vi "Loop_HW Camera.vi"() -> ()   [LabVIEW 2017, in "VisionSystem.lvlib"]
uses:
  VisionSystem.lvlib
  ENUM_HW_State.ctl
  Cluster_CMD to Vision.ctl
  Enum_ Field Targets.ctl
  ENUM_HW_Action.ctl
  Cluster_HW_Status.ctl
  <vilib>/vision/Image Controls.llb/IMAQ Image.ctl
  TypeDefs/Cluster_Camera Settings.ctl
  <vilib>/Rock Robotics/WPI/Camera/WPI_CameraImageSize.ctl
  <vilib>/Rock Robotics/WPI/Camera/WPI_CameraFrameRate.ctl
  <vilib>/Rock Robotics/WPI/Camera/WPI_CameraWhite Balance Values.ctl
  <vilib>/Rock Robotics/WPI/Camera/WPI_CameraExposure Values.ctl
  <vilib>/Rock Robotics/WPI/Camera/WPI_CameraDevRef.ctl
  Global_CMD Data.vi
  Globals/Global_STOP.vi
  Global_HW Status.vi
  <vilib>/vision/driver/NI_Vision_Acquisition_Software.lvlib
panel:
  in  "Clear error":bool
  in  "Reset Camera":bool
  in  "Reset Camera":bool
  out "cycle time (s)":dbl
  in  "Cam 1 Setings":T1={"Image Size"=enum."320x240", "Frame Rate (fps)"=35, "White Balance"=enum."Custom", "Exposure"=enum."Auto", "Exposure (%)"=0.0, "Brightness"=72, "Sharpness"=0, "Saturation"=0} {"Saturation" min=0 max=100 step=1; "Sharpness" min=0 max=100 step=1; "Brightness" min=0 max=100 step=1; "Exposure (%)" min=0.0 max=100.0 step=1.0}
  out "Error":errorcluster[](array[cluster])
  in  "Restore Settings":bool
  in  "Save Settings":bool
  in  "Cam 0 Setings":T1={"Image Size"=enum."320x240", "Frame Rate (fps)"=20, "White Balance"=enum."Auto", "Exposure"=enum."Auto", "Exposure (%)"=0.0, "Brightness"=0, "Sharpness"=0, "Saturation"=0} {"Saturation" min=0 max=100 step=1; "Sharpness" min=0 max=100 step=1; "Brightness" min=0 max=100 step=1; "Exposure (%)" min=0.0 max=100.0 step=1.0}
  out "Cam Array":T6(array[cluster]) {"BusType" format="%x"; "SerialNumberLow" format="%.0x"; "SerialNumberHigh" format="%.0x"}
  out "Image":T7(plugin-control)
  in  "Show Image":bool
  out "HW Status_OUT":T8 {"Cam Setings"."Saturation" min=0 max=100 step=1; "Cam Setings"."Sharpness" min=0 max=100 step=1; "Cam Setings"."Brightness" min=0 max=100 step=1; "Cam Setings"."Exposure (%)" min=0.0 max=100.0 step=1.0}
  out "Action":T11
  out "CMD_Camera":T12
  out "Current State":T13
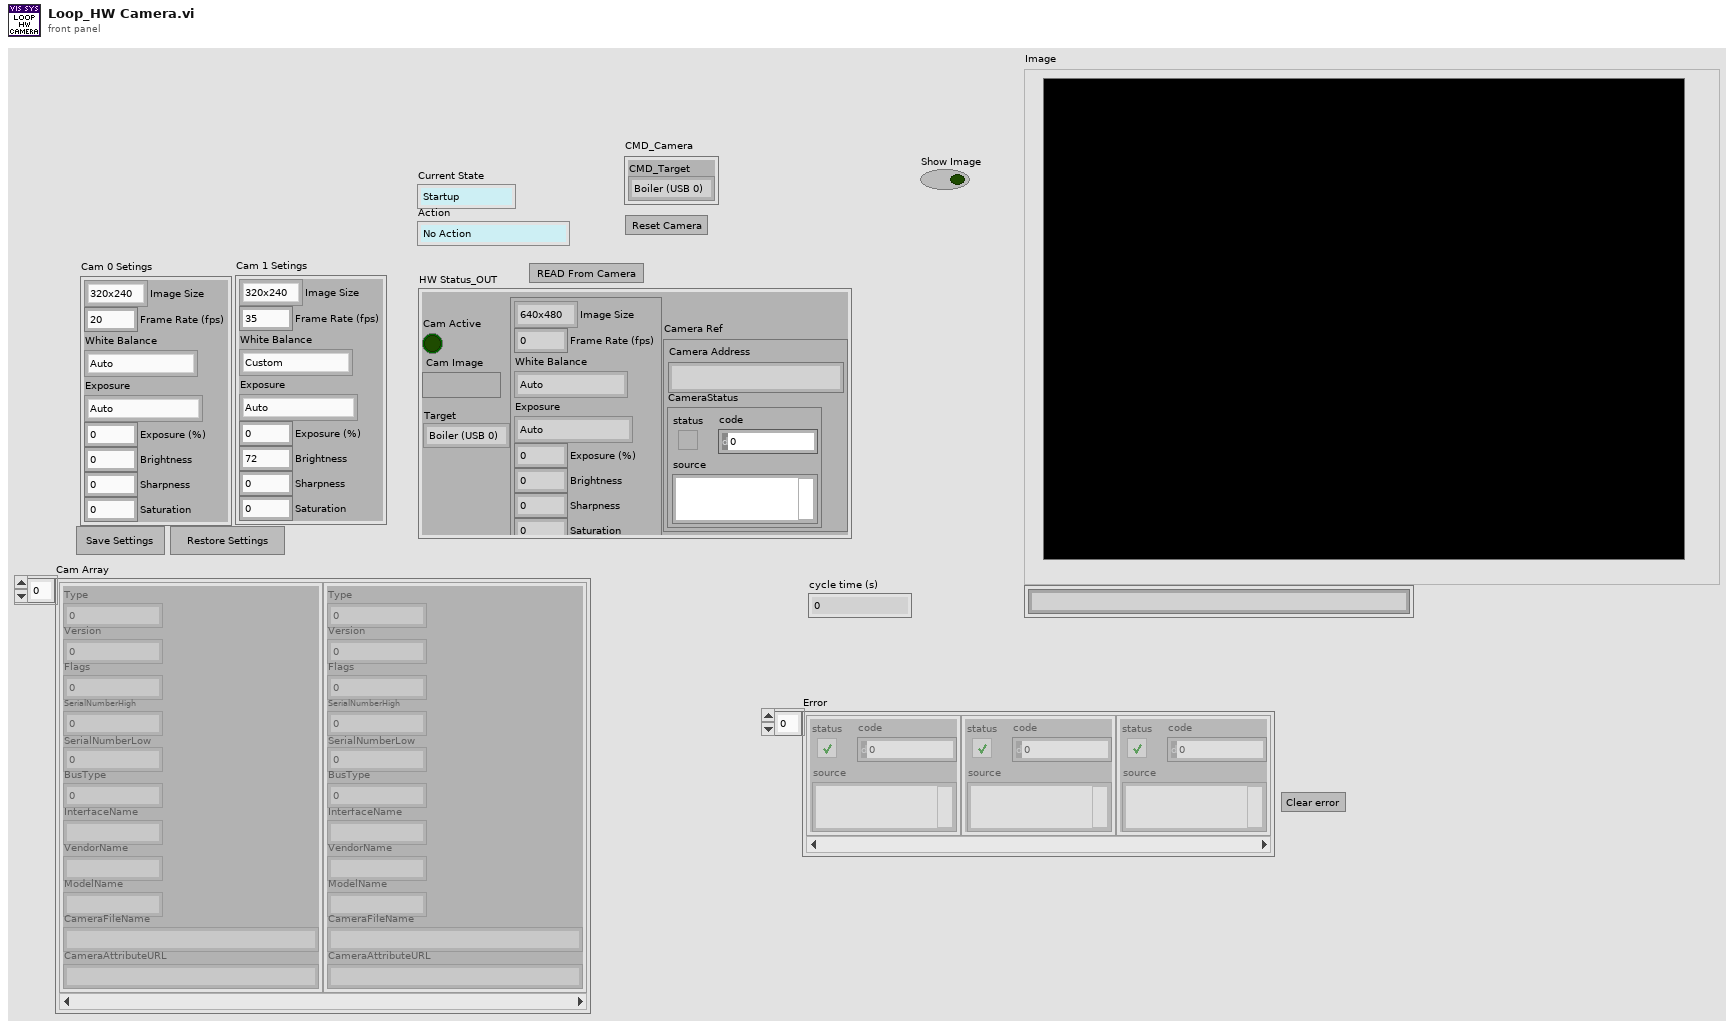
[diagram p1: front panel]
types:
  T1 = typedef "Cluster_Camera Settings.ctl" = cluster{"Image Size":T2, "Frame Rate (fps)":T3, "White Balance":T4, "Exposure":T5, "Exposure (%)":dbl, "Brightness":i32, "Sharpness":i32, "Saturation":i32}
  T2 = typedef "WPI_CameraImageSize.ctl" = enum16{"640x480", "320x240", "160x120", "Custom"}
  T3 = typedef "WPI_CameraFrameRate.ctl" = u32
  T4 = typedef "WPI_CameraWhite Balance Values.ctl" = enum16{"Auto", "Fixed indoor", "Fixed outdoor 1", "Fixed outdoor 2", "Fixed fluorescent 1", "Fixed fluorescent 2", "Hold current", "Custom"}
  T5 = typedef "WPI_CameraExposure Values.ctl" = enum16{"Auto", "Flicker-free 50 Hz", "Flicker-free 60 Hz", "Hold current", "Custom"}
  T6 = cluster{"Type":u32, "Version":u32, "Flags":u32, "SerialNumberHigh":u32, "SerialNumberLow":u32, "BusType":u32, "InterfaceName":string, "VendorName":string, "ModelName":string, "CameraFileName":string, "CameraAttributeURL":string}[]
  T7 = typedef "IMAQ Image.ctl" = refnum<image>
  T8 = typedef "VisionSystem.lvlib/Cluster_HW_Status.ctl" = cluster{"Cam Active":bool, "Cam Image":T7, "Cam Setings":T1, "Target":T9, "Camera Ref":T10}
  T9 = typedef "VisionSystem.lvlib/Enum_ Field Targets.ctl" = enum16{"Boiler (USB 0)", "Rope (USB 1)"}
  T10 = typedef "WPI_CameraDevRef.ctl" = cluster{"Camera Address":string, "CameraStatus":errorcluster}
  T11 = typedef "VisionSystem.lvlib/ENUM_HW_Action.ctl" = enum16{"No Action", "Reset Time", "Open Cam 0", "Open Cam 1", "Stop Camera", "Start Camera", "Acquire Camera", "Close Camera", "Read Avalable Cams", "Save Settings to File", "Restore Settings from File", "Open Image", "Close Image", "Set  Camera", "Read Cam Settings"}
  T12 = typedef "VisionSystem.lvlib/Cluster_CMD to Vision.ctl" = cluster{"CMD_Target":T9}
  T13 = typedef "VisionSystem.lvlib/ENUM_HW_State.ctl" = enum16{"Startup", "Idle", "Acquire", "Shutdown", "Setting"}
  T14 = cluster{"Actions":T11[], "State":T13, "Current Time":timestamp, "Start Time":timestamp, "Loop Time (ms)":u32, "CMD_HW":T12, "HW Status_OUT":T8, "Cam  Array":cluster{"Type":u32, "Version":u32, "Flags":u32, "SerialNumberHigh":u32, "SerialNumberLow":u32, "BusType":u32, "InterfaceName":string, "VendorName":string, "ModelName":string, "CameraFileName":string, "CameraAttributeURL":string}[], "Error ":errorcluster[], "Cam 0 Setings":T1, "Cam 1 Setings":T1, "Camera Readings":T1}
  T15 = typedef "Image Type" = u32
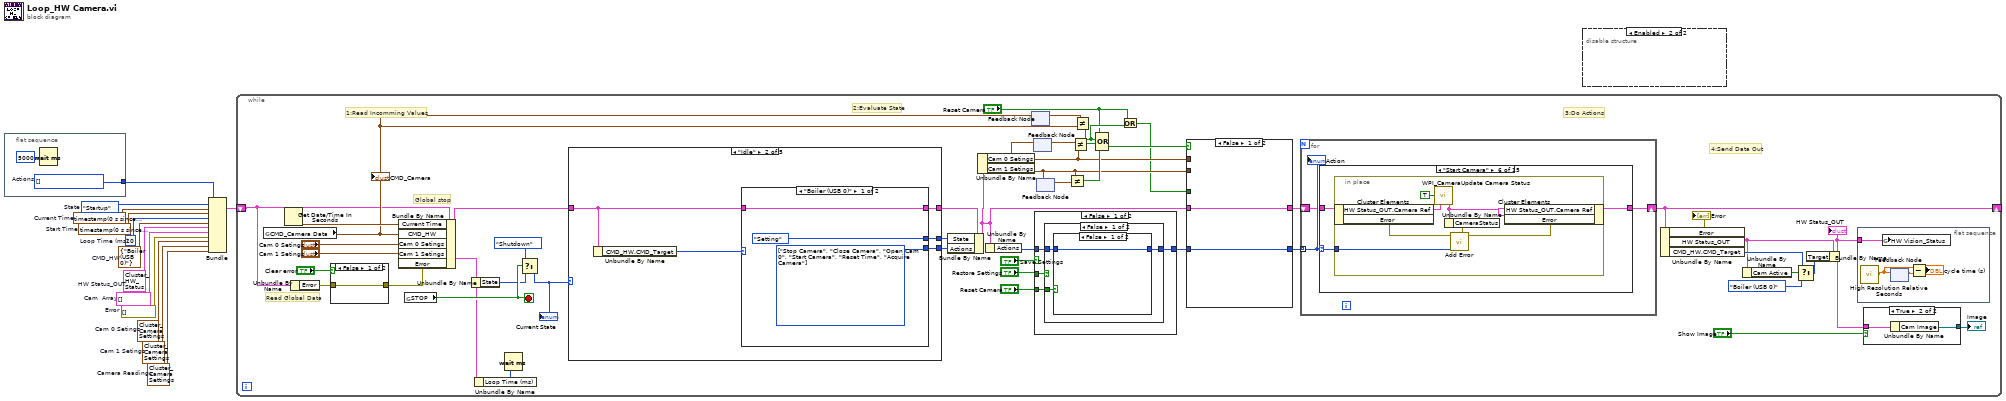
[diagram p0: block diagram]
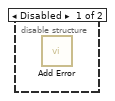
[diagram p2: hidden frame]
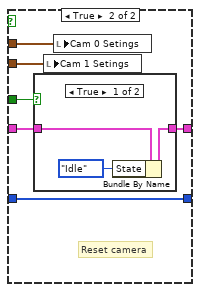
[diagram p4: hidden frame]
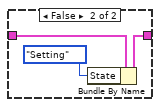
[diagram p5: hidden frame]
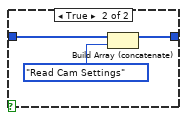
[diagram p6: hidden frame]
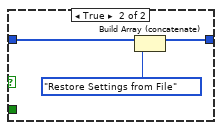
[diagram p7: hidden frame]
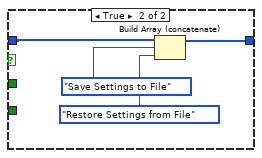
[diagram p8: hidden frame]
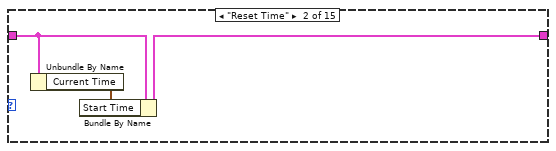
[diagram p11: hidden frame]
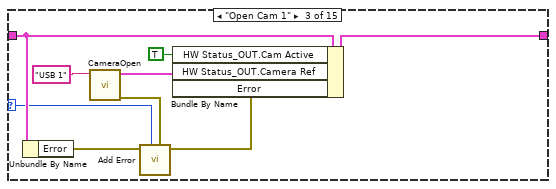
[diagram p12: hidden frame]
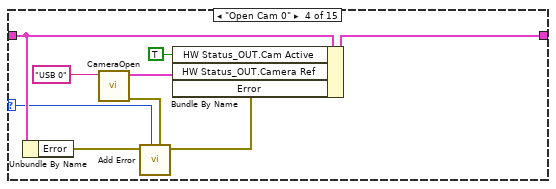
[diagram p13: hidden frame]
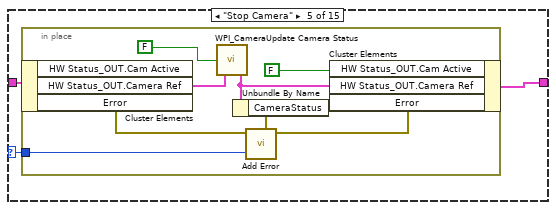
[diagram p14: hidden frame]
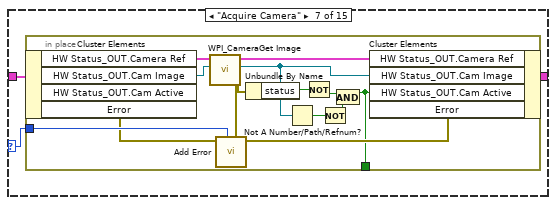
[diagram p15: hidden frame]
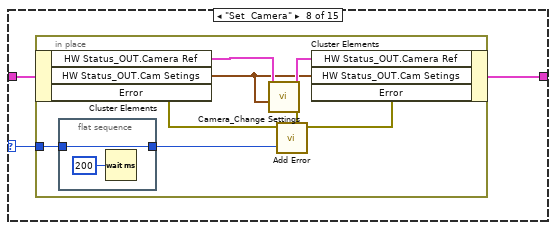
[diagram p16: hidden frame]
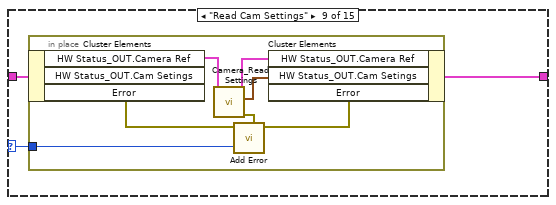
[diagram p17: hidden frame]
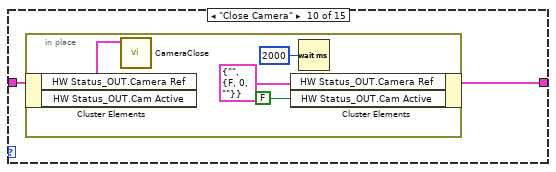
[diagram p18: hidden frame]
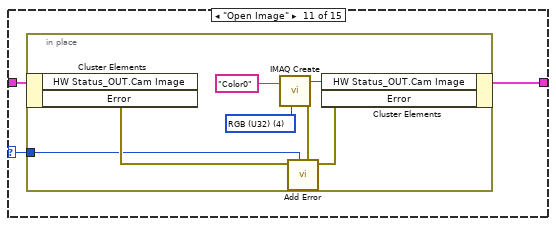
[diagram p19: hidden frame]
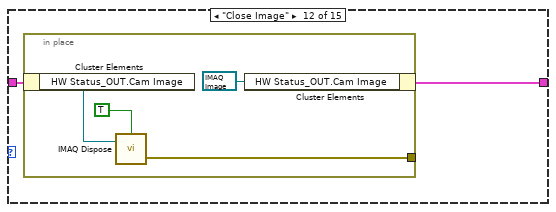
[diagram p20: hidden frame]
diagram:
  w1 = T1 {"Image Size"=enum."640x480", "Frame Rate (fps)"=20, "White Balance"=enum."Fixed fluorescent 1", "Exposure"=enum."Flicker-free 60 Hz", "Exposure (%)"=20.0, "Brightness"=0, "Sharpness"=0, "Saturation"=40}  # Camera Readings
  w2 = T1 {"Image Size"=enum."640x480", "Frame Rate (fps)"=0, "White Balance"=enum."Auto", "Exposure"=enum."Auto", "Exposure (%)"=0.0, "Brightness"=0, "Sharpness"=0, "Saturation"=0}  # Cam 1 Setings
  w3 = T1 {"Image Size"=enum."640x480", "Frame Rate (fps)"=0, "White Balance"=enum."Auto", "Exposure"=enum."Auto", "Exposure (%)"=0.0, "Brightness"=0, "Sharpness"=0, "Saturation"=0}  # Cam 0 Setings
  w4 = errorcluster[] []  # Error
  w5 = T6 []  # Cam  Array
  w6 = T8 {"Cam Active"=FALSE, "Cam Image"=refnum, "Cam Setings"={"Image Size"=enum."640x480", "Frame Rate (fps)"=0, "White Balance"=enum."Auto", "Exposure"=enum."Auto", "Exposure (%)"=0.0, "Brightness"=0, "Sharpness"=0, "Saturation"=0}, "Target"=enum."Boiler (USB 0)", "Camera Ref"={"Camera Address"="", "CameraStatus"={"status"=FALSE, "code"=0, "source"=""}}}  # HW Status_OUT
  w7 = T12 {"CMD_Target"=enum."Boiler (USB 0)"}  # CMD_HW
  w8 = u32 20  # Loop Time (ms)
  w10 = timestamp(0 s since 1904-01-01)  # Start Time
  w11 = timestamp(0 s since 1904-01-01)  # Current Time
  w12 = ENUM_HW_State."Startup"  # State
  n1 = flat-sequence {
    tunnel: [w15] -> w9
    frame #0 {
      w15 = T11[] [] items=["No Action", "Reset Time", "Open Cam 0", "Open Cam 1", "Stop Camera", "Start Camera", "Acquire Camera", "Close Camera", "Read Avalable Cams", "Save Settings to File", "Restore Settings from File", "Open Image", "Close Image", "Set  Camera", "Read Cam Settings"]  # Actions
      n2 = Wait (ms)(milliseconds to wait=u32 5000) -> ()  [unwired: 1 out]
    }
  }
  n3 = Bundle("Actions"=w9, "State"=w12, "Current Time"=w11, "Start Time"=w10, "Loop Time (ms)"=w8, "CMD_HW"=w7, "HW Status_OUT"=w6, "Cam  Array"=w5, "Error"=w4, "Cam 0 Setings"=w3, "Cam 1 Setings"=w2, "Camera Readings"=w1) -> (w13:T14)  [unwired: 1 in]
  n4 = while {
    shift-right: [w23] -> _
    shift-left: w13 -> [w22]
    stop <- w56 stop-if-true
    # "Read Global Data"
    # "1:Read Incomming Values"
    # "2:Evaluate State"
    # "3:Do Actions"
    # "4:Send Data Out"
    # "Global stop"
    n5 = global read "Global_CMD Data.vi" "CMD_Camera Data"() -> (w25:T12)
    "CMD_Camera" <- w25
    n6 = Get Date/Time In Seconds() -> (seconds since 1Jan1904=w60:timestamp)
    n7 = Unbundle By Name(w22) -> ("Error"=w20:errorcluster[])
    n8 = case shown="False" "Clear error" {
      tunnel: [w62 _] -> w19
      tunnel: w20 -> [w62 _]
      frame False {
      }
      frame True {
      }
    }
    n9 = Bundle By Name(cluster=w22, "Current Time"=w60, "CMD_HW"=w25, "Cam 0 Setings"="Cam 0 Setings", "Cam 1 Setings"="Cam 1 Setings", "Error"=w19) -> (w51:T14)
    n10 = global read "Global_Stop.vi" "STOP"() -> (w56:bool)
    n11 = Unbundle By Name(w51) -> ("State"=w54:T13)
    n12 = Unbundle By Name(w51) -> ("Loop Time (ms)"=w52:u32)
    n13 = Wait (ms)(milliseconds to wait=w52) -> ()  [unwired: 1 out]
    n14 = Select(t=ENUM_HW_State."Shutdown" ("State"), s=w56, f=w54) -> (s? t:f=w53:T13)
    "Current State" <- w53
    n15 = case shown="\"Idle\"" w53 {
      tunnel: w51 -> [w247 w251 w263 w291 w294]
      tunnel: [w247 w250 w262 w291 w294] -> w59
      tunnel: [ENUM_HW_State."Idle" ("State") w249 w261 ENUM_HW_State."Acquire" ("State") ENUM_HW_State."Shutdown" ("State")] -> w58
      tunnel: [w246 w248 w260 w289 w292] -> w57
      frame "Startup" {
        w246 = T11[] [enum."Read Avalable Cams", enum."Restore Settings from File", enum."Open Image", enum."Close Camera"] items=["No Action", "Reset Time", "Open Cam 0", "Open Cam 1", "Stop Camera", "Start Camera", "Acquire Camera", "Close Camera", "Read Avalable Cams", "Save Settings to File", "Restore Settings from File", "Open Image", "Close Image", "Set  Camera", "Read Cam Settings"] ("Actions")
      }
      frame "Idle" {
        n16 = Unbundle By Name(w251) -> ("CMD_HW.CMD_Target"=w252:T9)
        n17 = case shown="\"Boiler (USB 0)\"" w252 {
          tunnel: w251 -> [w253 w256]
          tunnel: [w253 w256] -> w250
          tunnel: [ENUM_HW_State."Setting" ("State") ENUM_HW_State."Setting" ("State")] -> w249
          tunnel: [w254 w257] -> w248
          frame "Boiler (USB 0)" {
            w254 = T11[] [enum."Stop Camera", enum."Close Camera", enum."Open Cam 0", enum."Start Camera", enum."Reset Time", enum."Acquire Camera"] items=["No Action", "Reset Time", "Open Cam 0", "Open Cam 1", "Stop Camera", "Start Camera", "Acquire Camera", "Close Camera", "Read Avalable Cams", "Save Settings to File", "Restore Settings from File", "Open Image", "Close Image", "Set  Camera", "Read Cam Settings"] ("Actions")
          }
          frame "Rope (USB 1)" {
            w257 = T11[] [enum."Stop Camera", enum."Close Camera", enum."Open Cam 1", enum."Start Camera", enum."Reset Time"] items=["No Action", "Reset Time", "Open Cam 0", "Open Cam 1", "Stop Camera", "Start Camera", "Acquire Camera", "Close Camera", "Read Avalable Cams", "Save Settings to File", "Restore Settings from File", "Open Image", "Close Image", "Set  Camera", "Read Cam Settings"] ("Actions")
          }
        }
      }
      frame "Setting" {
        n18 = Unbundle By Name(w263) -> ("HW Status_OUT.Cam Active"=w259:bool, "CMD_HW.CMD_Target"=w264:T9)
        n19 = case shown="False" w259 {
          tunnel: w264 -> [_ w278]
          tunnel: w263 -> [w273 w277]
          tunnel: [w273 w276] -> w262
          tunnel: [w265 w275] -> w261
          tunnel: [_ w274] -> w260
          frame False {
            n20 = Unbundle By Name(w273) -> ("Current Time"=w272:timestamp, "Start Time"=w271:timestamp)
            n21 = Subtract(x=w272, y=w271) -> (x-y=w270:dbl)
            n22 = Greater Or Equal?(x=w270, y=2.0) -> (x >= y?=w268:bool)
            n23 = Select(t=ENUM_HW_State."Idle" ("State"), s=w268, f=ENUM_HW_State."Setting" ("State")) -> (s? t:f=w265:T13)
          }
          frame True {
            n24 = case shown="\"Rope (USB 1)\"" w278 {
              tunnel: w277 -> [w282 w287]
              tunnel: [w281 w286] -> w276
              tunnel: [ENUM_HW_State."Acquire" ("State") ENUM_HW_State."Acquire" ("State")] -> w275
              tunnel: [w279 w284] -> w274
              frame "Rope (USB 1)" {
                w279 = T11[] [enum."Set  Camera", enum."Read Cam Settings", enum."Acquire Camera"] items=["No Action", "Reset Time", "Open Cam 0", "Open Cam 1", "Stop Camera", "Start Camera", "Acquire Camera", "Close Camera", "Read Avalable Cams", "Save Settings to File", "Restore Settings from File", "Open Image", "Close Image", "Set  Camera", "Read Cam Settings"] ("Actions")
                n25 = Unbundle By Name(w282) -> ("Cam 1 Setings"=w280:T1)
                n26 = Bundle By Name(cluster=w282, "HW Status_OUT.Cam Setings"=w280) -> (w281:T14)
              }
              frame "Boiler (USB 0)" {
                w284 = T11[] [enum."Set  Camera", enum."Read Cam Settings", enum."Acquire Camera"] items=["No Action", "Reset Time", "Open Cam 0", "Open Cam 1", "Stop Camera", "Start Camera", "Acquire Camera", "Close Camera", "Read Avalable Cams", "Save Settings to File", "Restore Settings from File", "Open Image", "Close Image", "Set  Camera", "Read Cam Settings"] ("Actions")
                n27 = Unbundle By Name(w287) -> ("Cam 0 Setings"=w285:T1)
                n28 = Bundle By Name(cluster=w287, "HW Status_OUT.Cam Setings"=w285) -> (w286:T14)
              }
            }
          }
        }
      }
      frame "Acquire" {
        w289 = T11[] [enum."Acquire Camera"] items=["No Action", "Reset Time", "Open Cam 0", "Open Cam 1", "Stop Camera", "Start Camera", "Acquire Camera", "Close Camera", "Read Avalable Cams", "Save Settings to File", "Restore Settings from File", "Open Image", "Close Image", "Set  Camera", "Read Cam Settings"] ("Actions")
      }
      frame "Shutdown" {
        w292 = T11[] [enum."Save Settings to File", enum."Stop Camera", enum."Close Camera", enum."Close Image"] items=["No Action", "Reset Time", "Open Cam 0", "Open Cam 1", "Stop Camera", "Start Camera", "Acquire Camera", "Close Camera", "Read Avalable Cams", "Save Settings to File", "Restore Settings from File", "Open Image", "Close Image", "Set  Camera", "Read Cam Settings"] ("Actions")
      }
    }
    n29 = Bundle By Name(cluster=w59, "State"=w58, "Actions"=w57) -> (w35:T14)
    n30 = Unbundle By Name(w35) -> ("Cam 0 Setings"=w27:T1, "Cam 1 Setings"=w28:T1)
    n31 = Unbundle By Name(w35) -> ("Actions"=w61:T11[])
    n32 = feedback #1() -> (w26:T12)  [unwired: 1 in]
    n33 = feedback-in #1(w25) -> ()
    n34 = feedback #2() -> (w42:T1)  [unwired: 1 in]
    n35 = feedback-in #2(w27) -> ()
    n36 = case shown="False" "Save Settings" {
      tunnel: w61 -> [w84 w98]
      tunnel: [w83 w97] -> w39
      tunnel: "Restore Settings" -> [w82 _]
      tunnel: "Reset Camera" -> [w81 _]
      frame False {
        n37 = case shown="False" w82 {
          tunnel: w84 -> [w86 w94]
          tunnel: [w85 w93] -> w83
          tunnel: w81 -> [w87 _]
          frame False {
            n38 = case shown="False" w87 {
              tunnel: w86 -> [w88 w91]
              tunnel: [w88 w90] -> w85
              frame False {
              }
              frame True {
                n39 = Build Array (concatenate)(w91, ENUM_HW_Action."Read Cam Settings" ("Action")) -> (w90:T11[])
              }
            }
          }
          frame True {
            n40 = Build Array (concatenate)(w94, ENUM_HW_Action."Restore Settings from File" ("Action")) -> (w93:T11[])
          }
        }
      }
      frame True {
        n41 = Build Array (concatenate)(w98, ENUM_HW_Action."Save Settings to File" ("Action"), ENUM_HW_Action."Restore Settings from File" ("Action")) -> (w97:T11[])
      }
    }
    n42 = feedback-in #3(w28) -> ()
    n43 = feedback #3() -> (w43:T1)  [unwired: 1 in]
    n44 = Not Equal?(x=w28, y=w43) -> (x != y?=w40:bool)
    n45 = Not Equal?(x=w42, y=w27) -> (x != y?=w41:bool)
    n46 = Not Equal?(x=w26, y=w25) -> (x != y?=w18:bool)
    n47 = Compound Arithmetic op=OR("Reset Camera", w18, w41, w40) -> (w37:bool)
    n48 = Or(x="Reset Camera", y=w18) -> (x .or. y?=w16:bool)
    n49 = case shown="False" w37 {
      tunnel: w39 -> [w68 w74]
      tunnel: [w68 w74] -> w38
      tunnel: [w67 w72] -> w36
      tunnel: w35 -> [w67 w73]
      tunnel: w28 -> [_ w71]
      tunnel: w27 -> [_ w70]
      tunnel: w16 -> [_ w69]
      frame False {
      }
      frame True {
        # "Reset camera"
        n50 = case shown="True" w69 {
          tunnel: w73 -> [w77 w80]
          tunnel: [w76 w79] -> w72
          frame True {
            n51 = Bundle By Name(cluster=w77, "State"=ENUM_HW_State."Idle") -> (w76:T14)
          }
          frame False {
            n52 = Bundle By Name(cluster=w80, "State"=ENUM_HW_State."Setting") -> (w79:T14)
          }
        }
        n53 = local write "Cam 1 Setings"(w71) -> ()
        n54 = local write "Cam 0 Setings"(w70) -> ()
      }
    }
    n55 = for {
      tunnel: w38 -> [w103] mode=indexing
      shift-right: [w102] -> w23
      shift-left: w36 -> [w101]
      n56 = case shown="\"Start Camera\"" w103 {
        selector: w103 -> [_ _ w111 w120 w126 w137 w149 w163 w176 _ w192 _ w208 w215 w230]
        tunnel: w101 -> [w104 w107 w113 w122 w128 w139 w148 w165 w178 w187 w194 w203 w212 w217 w232]
        tunnel: [w104 w106 w115 w124 w127 w138 w147 w164 w177 w186 w193 w202 w213 w216 w231] -> w102
        frame "No Action" {
        }
        frame "Reset Time" {
          n57 = Unbundle By Name(w107) -> ("Current Time"=w105:timestamp)
          n58 = Bundle By Name(cluster=w107, "Start Time"=w105) -> (w106:T14)
        }
        frame "Open Cam 1" {
          n59 = Unbundle By Name(w113) -> ("Error"=w112:errorcluster[])
          n60 = call "CameraOpen.vi"("Camera Address"="USB 1" ("format string")) -> ("error out"=w109:errorcluster, "CameraDevRef"=w114:T10)  [unwired: 1 in, 8 out]
          n61 = call "Add Error.vi"("Error"=w109, "Action"=w111, "Error list"=w112) -> ("Error list Out"=w110:errorcluster[])  [unwired: 8 in]
          n62 = Bundle By Name(cluster=w113, "HW Status_OUT.Cam Active"=TRUE, "HW Status_OUT.Camera Ref"=w114, "Error"=w110) -> (w115:T14)
        }
        frame "Open Cam 0" {
          n63 = Unbundle By Name(w122) -> ("Error"=w121:errorcluster[])
          n64 = call "CameraOpen.vi"("Camera Address"="USB 0" ("format string")) -> ("error out"=w118:errorcluster, "CameraDevRef"=w123:T10)  [unwired: 1 in, 8 out]
          n65 = call "Add Error.vi"("Error"=w118, "Action"=w120, "Error list"=w121) -> ("Error list Out"=w119:errorcluster[])  [unwired: 8 in]
          n66 = Bundle By Name(cluster=w122, "HW Status_OUT.Cam Active"=TRUE, "HW Status_OUT.Camera Ref"=w123, "Error"=w119) -> (w124:T14)
        }
        frame "Stop Camera" {
          n67 = in-place {
            in-place-border: w126 -> [w134]
            n68 = in-place-cluster #4(w128) -> ("HW Status_OUT.Camera Ref"=w135:T10, "Error"=w133:errorcluster[])  [unwired: 1 out]
            n69 = call <vilib>:"WPI_CameraUpdate Camera Status.vi"("CameraDevRef In"=w135, "Enable Vision"=FALSE) -> ("CameraDevRef Out"=w131:T10)  [unwired: 3 in]
            n70 = Unbundle By Name(w131) -> ("CameraStatus"=w130:errorcluster)
            n71 = call "Add Error.vi"("Error"=w130, "Action"=w134, "Error list"=w133) -> ("Error list Out"=w132:errorcluster[])  [unwired: 8 in]
            n72 = in-place-cluster #4("HW Status_OUT.Cam Active"=FALSE, "HW Status_OUT.Camera Ref"=w131, "Error"=w132) -> (w127:T14)
          }
        }
        frame "Start Camera" {
          n73 = in-place {
            in-place-border: w137 -> [w144]
            n74 = in-place-cluster #5(w139) -> ("HW Status_OUT.Camera Ref"=w145:T10, "Error"=w143:errorcluster[])
            n75 = call <vilib>:"WPI_CameraUpdate Camera Status.vi"("CameraDevRef In"=w145, "Enable Vision"=TRUE) -> ("CameraDevRef Out"=w141:T10)  [unwired: 3 in]
            n76 = Unbundle By Name(w141) -> ("CameraStatus"=w140:errorcluster)
            n77 = call "Add Error.vi"("Error"=w140, "Action"=w144, "Error list"=w143) -> ("Error list Out"=w142:errorcluster[])  [unwired: 8 in]
            n78 = in-place-cluster #5("HW Status_OUT.Camera Ref"=w141, "Error"=w142) -> (w138:T14)
          }
        }
        frame "Acquire Camera" {
          n79 = in-place {
            in-place-border: w149 -> [w159]
            in-place-border: [w150] -> _
            n80 = in-place-cluster #6(w148) -> ("HW Status_OUT.Camera Ref"=w162:T10, "HW Status_OUT.Cam Image"=w160:T7, "Error"=w158:errorcluster[])  [unwired: 1 out]
            n81 = call <vilib>:"WPI_CameraGet Image.vi"("Image"=w160, "CameraDevRef"=w162) -> ("error out"=w156:errorcluster, "Image Out"=w153:T7, "CameraDevRef Out"=w161:T10)  [unwired: 7 in]
            n82 = call "Add Error.vi"("Error"=w156, "Action"=w159, "Error list"=w158) -> ("Error list Out"=w157:errorcluster[])  [unwired: 8 in]
            n83 = Unbundle By Name(w156) -> ("status"=w155:bool)
            n84 = Not A Number/Path/Refnum?(number/path/refnum=w153) -> (NaN/Path/Refnum?=w152:bool)
            n85 = Not(x=w155) -> (.not. x?=w154:bool)
            n86 = Not(x=w152) -> (.not. x?=w151:bool)
            n87 = And(x=w154, y=w151) -> (x .and. y?=w150:bool)
            n88 = in-place-cluster #6("HW Status_OUT.Camera Ref"=w161, "HW Status_OUT.Cam Image"=w153, "HW Status_OUT.Cam Active"=w150, "Error"=w157) -> (w147:T14)
          }
        }
        frame "Set  Camera" {
          n89 = in-place {
            in-place-border: w163 -> [w167]
            n90 = in-place-cluster #7(w165) -> ("HW Status_OUT.Camera Ref"=w171:T10, "HW Status_OUT.Cam Setings"=w168:T1, "Error"=w173:errorcluster[])
            n91 = flat-sequence {
              tunnel: [w174] -> w166
              tunnel: w167 -> [w174]
              frame #0 {
                n92 = Wait (ms)(milliseconds to wait=u32 200) -> ()  [unwired: 1 out]
              }
            }
            n93 = call "Camera_Change Settings.vi"("Camera Settings"=w168, "CameraDevRef"=w171) -> ("Error Out"=w169:errorcluster, "CameraDevRef Out"=w170:T10)  [unwired: 8 in]
            n94 = call "Add Error.vi"("Error"=w169, "Action"=w166, "Error list"=w173) -> ("Error list Out"=w172:errorcluster[])  [unwired: 8 in]
            n95 = in-place-cluster #7("HW Status_OUT.Camera Ref"=w170, "HW Status_OUT.Cam Setings"=w168, "Error"=w172) -> (w164:T14)
          }
        }
        frame "Read Cam Settings" {
          n96 = in-place {
            in-place-border: w176 -> [w185]
            n97 = in-place-cluster #8(w178) -> ("HW Status_OUT.Camera Ref"=w182:T10, "Error"=w184:errorcluster[])  [unwired: 1 out]
            n98 = call "Camera_Read Settings.vi"("CameraDevRef"=w182) -> ("Error Out"=w180:errorcluster, "Camera Settings"=w179:T1, "CameraDevRef Out"=w181:T10)  [unwired: 8 in]
            n99 = call "Add Error.vi"("Error"=w180, "Action"=w185, "Error list"=w184) -> ("Error list Out"=w183:errorcluster[])  [unwired: 8 in]
            n100 = in-place-cluster #8("HW Status_OUT.Camera Ref"=w181, "HW Status_OUT.Cam Setings"=w179, "Error"=w183) -> (w177:T14)
          }
        }
        frame "Close Camera" {
          n101 = in-place {
            n102 = in-place-cluster #9(w187) -> ("HW Status_OUT.Camera Ref"=w191:T10)  [unwired: 1 out]
            n103 = call "CameraClose.vi"("CameraDevRef"=w191) -> ()  [unwired: 10 in, 1 out]
            n104 = in-place-cluster #9("HW Status_OUT.Camera Ref"=T10 {"Camera Address"="", "CameraStatus"={"status"=FALSE, "code"=0, "source"=""}} ("Cam Ref"), "HW Status_OUT.Cam Active"=FALSE) -> (w186:T14)
            n105 = Wait (ms)(milliseconds to wait=u32 2000) -> ()  [unwired: 1 out]
          }
        }
        frame "Open Image" {
          n106 = in-place {
            in-place-border: w192 -> [w195]
            w201 = T15 4 items=["Grayscale (U8)", "Grayscale (I16)", "Grayscale (SGL)", "Complex (CSG)", "RGB (U32)", "HSL (U32)", "RGB (U64)", "Grayscale (U16)"] ("Image Type")
            n107 = in-place-cluster #10(w194) -> ("Error"=w198:errorcluster[])  [unwired: 1 out]
            n108 = call "IMAQ Create"("Image Name"="Color0", "Image Type"=w201) -> ("New Image"=w199:T7, "error out"=w196:errorcluster)  [unwired: 2 in, 1 out]
            n109 = call "Add Error.vi"("Error"=w196, "Action"=w195, "Error list"=w198) -> ("Error list Out"=w197:errorcluster[])  [unwired: 8 in]
            n110 = in-place-cluster #10("HW Status_OUT.Cam Image"=w199, "Error"=w197) -> (w193:T14)
          }
        }
        frame "Close Image" {
          n111 = in-place {
            in-place-border: [w204] -> _
            n112 = in-place-cluster #11(w203) -> ("HW Status_OUT.Cam Image"=w206:T7)
            n113 = call "IMAQ Dispose"("All Images? (No)"=TRUE, "Image"=w206) -> ("error out"=w204:errorcluster)  [unwired: 4 in]
            n114 = in-place-cluster #11("HW Status_OUT.Cam Image"=T7 refnum) -> (w202:T14)
          }
        }
        frame "Read Avalable Cams" {
          n115 = Unbundle By Name(w212) -> ("Error"=w211:errorcluster[])
          n116 = call <vilib>:"IMAQdx Enumerate Cameras.vi"() -> ("error out"=w209:errorcluster, "Camera Information Array"=w214:T6)  [unwired: 10 in]
          "Cam Array" <- w214
          n117 = call "Add Error.vi"("Error"=w209, "Action"=w208, "Error list"=w211) -> ("Error list Out"=w210:errorcluster[])  [unwired: 8 in]
          n118 = Bundle By Name(cluster=w212, "Cam  Array"=w214, "Error"=w210) -> (w213:T14)
        }
        frame "Save Settings to File" {
          n119 = in-place {
            in-place-border: w215 -> [w218]
            w224 = TRUE ("Read(f)Write(t)")
            n120 = in-place-cluster #12(w217) -> ("Cam 0 Setings"=w227:T1, "Cam 1 Setings"=w223:T1, "Error"=w221:errorcluster[])
            n121 = call "Read-Write Camera Settings to File.vi"("Read(f)Write(t)"=w224, "Cam ID"=u8 1, "Cam Setings"=w223) -> ("Error Out"=w228:errorcluster, "Cam Setings Out"=w222:T1)  [unwired: 6 in, 1 out]
            n122 = call "Read-Write Camera Settings to File.vi"("Read(f)Write(t)"=w224, "Cam ID"=u8 0, "Error"=w228, "Cam Setings"=w227) -> ("Error Out"=w219:errorcluster, "Cam Setings Out"=w226:T1)  [unwired: 5 in, 1 out]
            n123 = call "Add Error.vi"("Error"=w219, "Action"=w218, "Error list"=w221) -> ("Error list Out"=w220:errorcluster[])  [unwired: 8 in]
            n124 = in-place-cluster #12("Cam 0 Setings"=w226, "Cam 1 Setings"=w222, "Error"=w220) -> (w216:T14)
          }
        }
        frame "Restore Settings from File" {
          n125 = in-place {
            in-place-border: w230 -> [w233]
            w239 = FALSE ("Read(f)Write(t)")
            n126 = in-place-cluster #13(w232) -> ("Cam 0 Setings"=w242:T1, "Cam 1 Setings"=w238:T1, "Error"=w236:errorcluster[])
            n127 = call "Read-Write Camera Settings to File.vi"("Read(f)Write(t)"=w239, "Cam ID"=u8 1, "Cam Setings"=w238) -> ("Error Out"=w243:errorcluster, "Cam Setings Out"=w237:T1)  [unwired: 6 in, 1 out]
            n128 = call "Read-Write Camera Settings to File.vi"("Read(f)Write(t)"=w239, "Cam ID"=u8 0, "Error"=w243, "Cam Setings"=w242) -> ("Error Out"=w234:errorcluster, "Cam Setings Out"=w241:T1)  [unwired: 5 in, 1 out]
            n129 = call "Add Error.vi"("Error"=w234, "Action"=w233, "Error list"=w236) -> ("Error list Out"=w235:errorcluster[])  [unwired: 8 in]
            n130 = in-place-cluster #13("Cam 0 Setings"=w241, "Cam 1 Setings"=w237, "Error"=w235) -> (w231:T14)
          }
        }
      }
      "Action" <- w103
    }
    n131 = Unbundle By Name(w23) -> ("Error"=→"Error":errorcluster[], "HW Status_OUT"=w32:T8, "CMD_HW.CMD_Target"=w33:T9)
    n132 = Unbundle By Name(w32) -> ("Cam Active"=w34:bool)
    n133 = Select(t=w33, s=w34, f=Enum__Field_Targets."Boiler (USB 0)") -> (s? t:f=w30:T9)
    n134 = Bundle By Name(cluster=w32, "Target"=w30) -> (w31:T8)
    "HW Status_OUT" <- w31
    n135 = flat-sequence {
      tunnel: w31 -> [w66]
      frame #0 {
        n136 = call <vilib>:"High Resolution Relative Seconds.vi"() -> ("relative seconds"=w64:dbl)
        n137 = global write "Global_HW Status.vi" "HW Vision_Status"(w66) -> ()
        n138 = feedback-in #14(w64) -> ()
        n139 = feedback #14() -> (w65:dbl)  [unwired: 1 in]
        n140 = Subtract(x=w64, y=w65) -> (x-y=→"cycle time (s)":dbl)
      }
    }
    n141 = case shown="True" "Show Image" {
      tunnel: w31 -> [_ w100]
      tunnel: [_ w99] -> w49
      frame False {
      }
      frame True {
        n142 = Unbundle By Name(w100) -> ("Cam Image"=w99:T7)
      }
    }
    "Image" <- w49
  }
  n143 = disable-structure shown="Enabled" {
    frame Disabled {
      n144 = call "Add Error.vi"() -> ()  [unwired: 11 in, 1 out]
    }
    frame Enabled {
    }
  }
